vi "Calculate DIDPID Frame Length.vi"(11 "PID In":T1 {"Signals"."Byte Order" items=["Little Endian", "Big Endian"]; "Signals"."Data Type" items=["Signed", "Unsigned", "IEEE Float"]}) -> (3 "Frame Length":u8)   [LabVIEW 2015, in "Diagnostics Addon Shared.lvlib"]
uses:
  Diagnostics Addon Shared.lvlib
  DIDPID Parameters.ctl
  DIDPID Signal Parameters.ctl
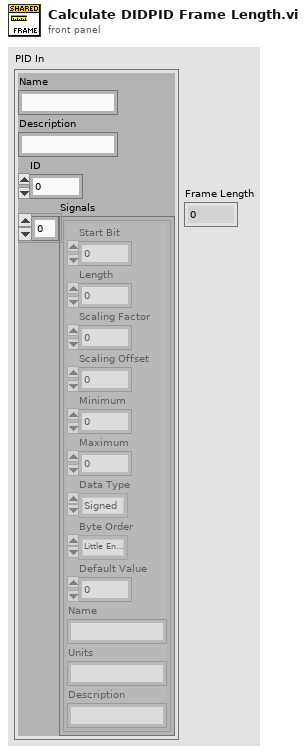
[diagram p1: front panel]
types:
  T1 = typedef "Diagnostics Addon Shared.lvlib/DIDPID Parameters.ctl" = cluster{"Name":string, "Description":string, "ID":u16, "Signals":T2[]}
  T2 = typedef "Diagnostics Addon Shared.lvlib/DIDPID Signal Parameters.ctl" = cluster{"Start Bit":u8, "Length":u8, "Scaling Factor":dbl, "Scaling Offset":dbl, "Minimum":dbl, "Maximum":dbl, "Data Type":u32, "Byte Order":u32, "Default Value":dbl, "Name":string, "Units":string, "Description":string}
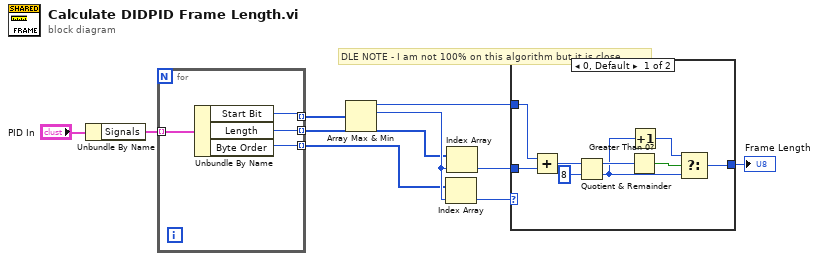
[diagram p0: block diagram]
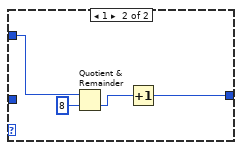
[diagram p2: hidden frame]
diagram:
  # "DLE NOTE - I am not 100% on this algorithm but it is close."
  n1 = Unbundle By Name("PID In") -> ("Signals"=w1:T2[])
  n2 = for {
    tunnel: w1 -> [w14] mode=indexing
    tunnel: [w13] -> w3 mode=indexing
    tunnel: [w12] -> w4 mode=indexing
    tunnel: [w11] -> w5 mode=indexing
    n3 = Unbundle By Name(w14) -> ("Start Bit"=w13:u8, "Length"=w12:u8, "Byte Order"=w11:u32)
  }
  n4 = Array Max & Min(array=w3) -> (max value=w8:u8, max index (indices)=w6:i32)  [unwired: 2 out]
  n5 = Index Array(array=w5, index=w6) -> (element=w7:u32)
  n6 = Index Array(array=w4, index=w6) -> (element=w9:u8)
  n7 = case shown="0, Default" w7 {
    tunnel: w8 -> [w23 w24]
    tunnel: w9 -> [w22 _]
    tunnel: [w15 w25] -> w10
    frame 0, Default {
      n8 = Add(x=w23, y=w22) -> (x+y=w21:u8)
      n9 = Quotient & Remainder(x=w21, y=u8 8) -> (x-y*floor(x/y)=w19:u8, floor(x/y)=w17:u8)
      n10 = Greater Than 0?(x=w19) -> (x > 0?=w18:bool)
      n11 = Increment(x=w17) -> (x+1=w16:u8)
      n12 = Select(t=w16, s=w18, f=w17) -> (s? t:f=w15:u8)
    }
    frame 1 {
      n13 = Quotient & Remainder(x=w24, y=u8 8) -> (floor(x/y)=w26:u8)  [unwired: 1 out]
      n14 = Increment(x=w26) -> (x+1=w25:u8)
    }
  }
  "Frame Length" <- w10
